vi "error_handler.vi"(7 "calling_vi":refnum<vi>, 8 "error in (no error)":errorcluster, 10 "ni.com link visible (F)":bool, 11 "type of dialog (OK msg:1)":T1=enum."OK message") -> (0 "error out":errorcluster)   [LabVIEW 2015, in "lv-dialog.lvlib"]
doc: "Indicates whether an error occurred. If an error occurred, this VI returns a description of the error and optionally displays a dialog box."
uses:
  lv-dialog.lvlib
  <vilib>/Utility/error.llb/DialogTypeEnum.ctl
  <vilib>/Utility/error.llb/whitespace.ctl
  api/v1/public/_controls/selection.ctl
  api/v1/public/class/v1.lvclass
  api/v1/v1.lvlib
panel:
  # "reinitialize to default to display instructions"
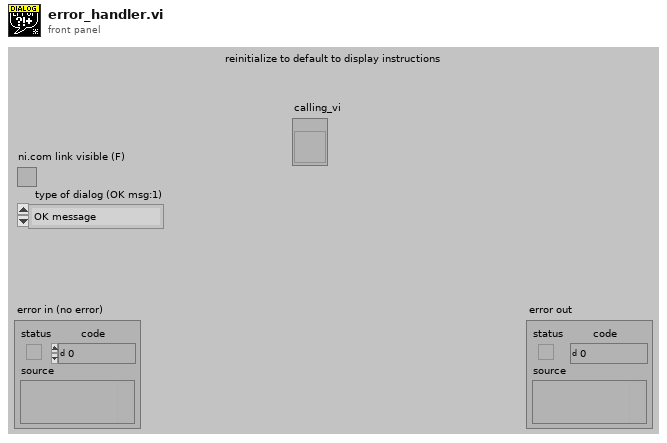
[diagram p1: front panel]
types:
  T1 = typedef "DialogTypeEnum.ctl" = enum16{"no dialog", "OK message", "continue or stop message", "auto error handling dialog", "OK message + warnings", "continue/stop + warnings"}
  T2 = cluster{"Error %d occurred at %s":string, "Warning %d occurred at %s":string, "Possible reasons: %s":string, "Error not listed":string, "GetCommError x%lx":string, "Continue":string, "Stop":string, "an unidentified location":string, "No Error":string, "Help":string}
  T3 = typedef "lv-dialog.lvlib/v1.lvlib/selection.ctl" = enum16{"null", "panel_closed", "button_1", "button_2", "button_3", "cancelled"}
  T4 = typedef "TagReturnType.ctl" = enum16{"No Tag", "<err>", "<append>"}
  T5 = typedef "whitespace.ctl" = u16
  T6 = cluster{"message":string, "Continue":string, "Stop":string}
  T7 = cluster{"ni.com link visible (F)":bool, "code":i32, "Bold Length":i32[], "Bold Start":i32[], "Source Out":string, "Details Out":string, "type of dialog (OK msg:1)":T1, bool, "Continue":string, "Stop":string, "Continue":string, "Tag Found?":T4}
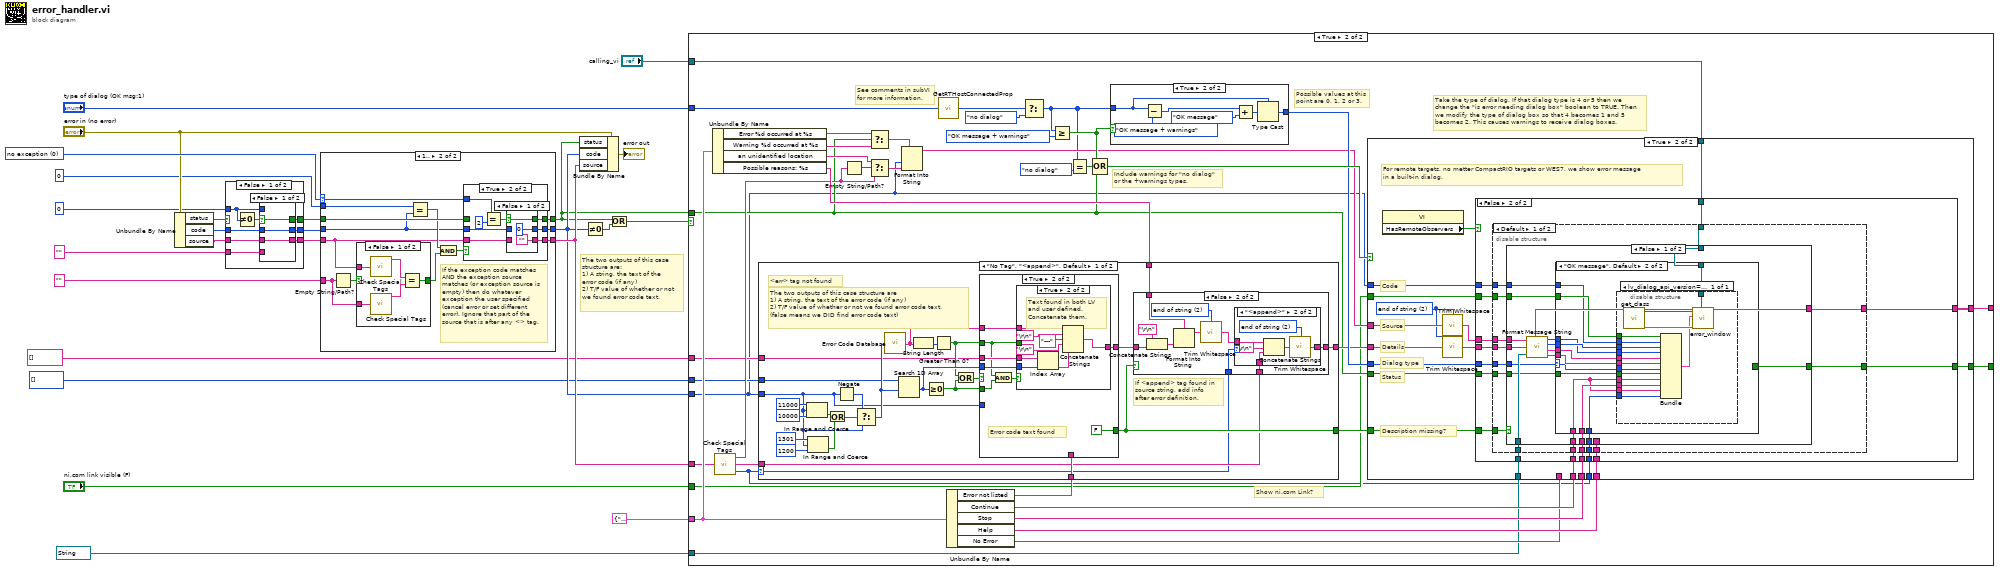
[diagram p0: block diagram]
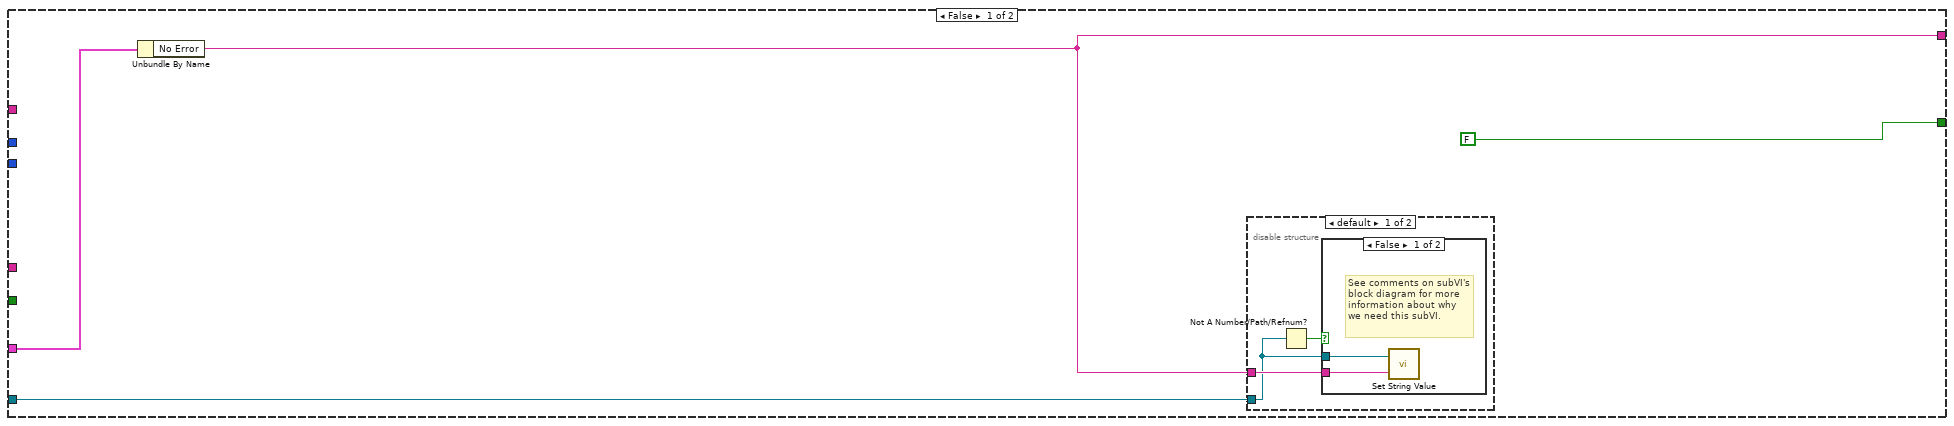
[diagram p8: hidden frame]
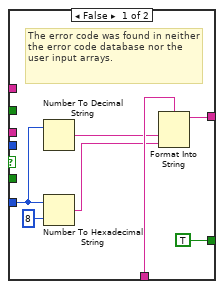
[diagram p14: hidden frame]
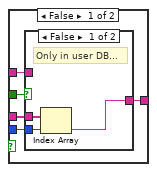
[diagram p15: hidden frame]
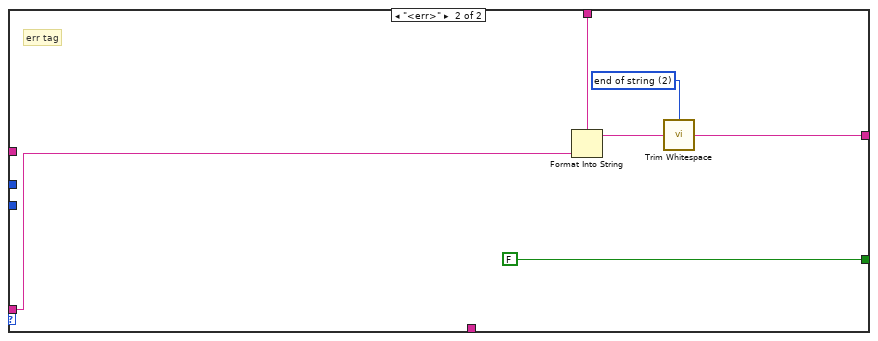
[diagram p17: hidden frame]
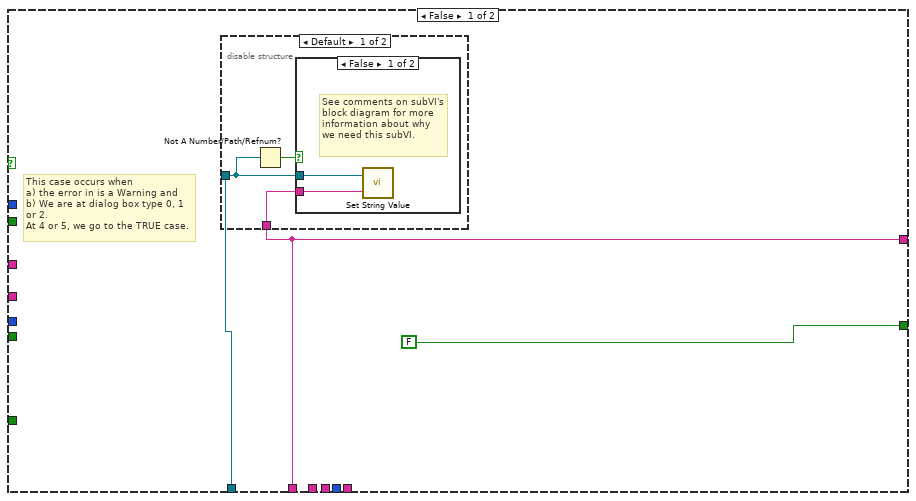
[diagram p18: hidden frame]
diagram:
  w20 = 0 items=["no exception", "cancel error on match", "set error on match"] ("[exception action] (none:0)")
  # "The two outputs of this case structure are:\n1) A string, the text of the error code (if any)\n2) T/F value of whether or not we found error code text."
  n1 = Unbundle By Name("error in (no error)") -> ("status"=w8:bool, "code"=w21:i32, "source"=w25:string)
  n2 = case shown="False" w8 {
    selector: w8 -> [_ w42]
    tunnel: [w31 w41] -> w23
    tunnel: [w32 w42] -> w22
    tunnel: w21 -> [w28 w41]
    tunnel: [w30 w40] -> w24
    tunnel: w25 -> [w29 w40]
    tunnel: 0 ("[error code] (0)") -> [w27 _]
    tunnel: "" ("[error source] (\" \")") -> [w26 _]
    frame False {
      n3 = Not Equal To 0?(x=w27) -> (x != 0?=w33:bool)
      n4 = case shown="False" w33 {
        selector: w33 -> [w36 w39]
        tunnel: [w36 w39] -> w32
        tunnel: w27 -> [_ w38]
        tunnel: [w34 w38] -> w31
        tunnel: w26 -> [_ w37]
        tunnel: [w35 w37] -> w30
        tunnel: w29 -> [w35 _]
        tunnel: w28 -> [w34 _]
        frame False {
        }
        frame True {
        }
      }
    }
    frame True {
    }
  }
  n5 = case shown="1.." w20 {
    selector: w20 -> [_ w50]
    tunnel: [w45 w58] -> w4
    tunnel: w22 -> [w45 w56]
    tunnel: [w44 w57] -> w9
    tunnel: w23 -> [w44 w54]
    tunnel: [w43 w52] -> w18
    tunnel: w24 -> [w43 w48]
    tunnel: 0 ("[exception code]") -> [_ w51]
    tunnel: "" ("[exception source]") -> [_ w47]
    frame ..0 {
    }
    frame 1.. {
      # "If the exception code matches AND the exception source matches (or exception source is empty) then do whatever exception the user specified (cancel error or set different error). Ignore that part of the source that is after any <> tag."
      n6 = Empty String/Path?(string/path=w47) -> (empty?=w49:bool)
      n7 = case shown="False" w49 {
        selector: w49 -> [_ w64]
        tunnel: w48 -> [w63 _]
        tunnel: w47 -> [w62 _]
        tunnel: [w61 w64] -> w46
        frame False {
          n8 = call <vilib>:"Check Special Tags.vi"("source"=w63) -> ("Before Tag (source)"=w60:string)  [unwired: 2 out]
          n9 = call <vilib>:"Check Special Tags.vi"("source"=w62) -> ("Before Tag (source)"=w59:string)  [unwired: 2 out]
          n10 = Equal?(x=w60, y=w59) -> (x = y?=w61:bool)
        }
        frame True {
          # "Empty string always matches."
        }
      }
      n11 = Equal?(x=w51, y=w54) -> (x = y?=w55:bool)
      n12 = And(x=w55, y=w46) -> (x .and. y?=w53:bool)
      n13 = case shown="True" w53 {
        tunnel: [w67 w68] -> w58
        tunnel: [w66 w72] -> w57
        tunnel: w56 -> [w67 _]
        tunnel: w54 -> [w66 w71]
        tunnel: w50 -> [_ w75]
        tunnel: [w65 w70] -> w52
        tunnel: w48 -> [w65 w69]
        frame False {
        }
        frame True {
          n14 = Equal?(x=w75, y=2) -> (x = y?=w73:bool)
          n15 = case shown="False" w73 {
            selector: w73 -> [w78 w81]
            tunnel: [0 w80] -> w72
            tunnel: w71 -> [_ w80]
            tunnel: ["" ("Empty String Constant") w79] -> w70
            tunnel: w69 -> [_ w79]
            tunnel: [w78 w81] -> w68
            frame False {
            }
            frame True {
            }
          }
        }
      }
    }
  }
  n16 = Bundle By Name(cluster="error in (no error)", "status"=w4, "code"=w9, "source"=w18) -> (→"error out":errorcluster)
  n17 = Not Equal To 0?(x=w9) -> (x != 0?=w3:bool)
  n18 = Or(x=w4, y=w3) -> (x .or. y?=w19:bool)
  n19 = case shown="True" w19 {
    tunnel: [w83 w112] -> _
    tunnel: w4 -> [_ w95]
    tunnel: w18 -> [_ w102]
    tunnel: T2 {"Error %d occurred at %s"="Error %d occurred at %s", "Warning %d occurred at %s"="Warning %d occurred at %s", "Possible reasons: %s"="<b>Possible reason(s):</b>\\n%s", "Error not listed"="This error code is undefined. Undefined errors might occur for a number of reasons. For example, no one has provided a description for the code, or you might have wired a number that is not an error code to the error code input. \n\nAdditionally, undefined error codes might occur because the error relates to a third-party object, such as the operating system or ActiveX. For these third-party errors, you might be able to obtain a description of the error by searching the Web for the error code (%s) or for its hexadecimal representation (0x%s).", "GetCommError x%lx"="Windows GetCommError:  The hex value of this code is <B>x%04lx</B>.\n\nInterpret it bit-wise as follows:\n<B>x4000</B>: serial port VI error\n<B>x0001</B>: receiving queue overflowed or character was received after end-of-file character\n<B>x0002</B>: character was lost by overwrite\n<B>x0004</B>: parity error\n<B>x0008</B>: framing error\n<B>x0010</B>: break condition\n<B>x0020</B>: CTS timeout\n<B>x0040</B>: DSR timeout\n<B>x0080</B>: RLSD timeout\n<B>x0100</B>: transmission queue was full when new character arrived\n<B>x0200</B>: parallel device timeout\n<B>x0400</B>: parallel device I/O error\n<B>x0800</B>: parallel device not selected\n<B>x1000</B>: parallel device out of paper\n<B>x8000</B>: requested mode is  not supported or the idComDev parameter is invalid.", "Continue"="Continue", "Stop"="Stop", "an unidentified location"="an unidentified location", "No Error"="No Error", "Help"="Why not found?"} ("prompts") -> [w85 w120]
    tunnel: [FALSE ("Stop 2") w115] -> _
    tunnel: refnum<vi> refnum ("String to Format (not a refnum)") -> [w82 w108]
    tunnel: w9 -> [_ w93]
    tunnel: string[] [] ("[user-defined descriptions]") -> [_ w99]
    tunnel: i32[] [] ("[user-defined codes]") -> [_ w98]
    tunnel: "type of dialog (OK msg:1)" -> [_ w97]
    tunnel: "ni.com link visible (F)" -> [_ w94]
    tunnel: "calling_vi" -> [_ w91]
    frame False {
      n20 = Unbundle By Name(w85) -> ("No Error"=w83:string)
      n21 = disable-structure shown="default" {
        disable-tunnel: w83 -> [w88 _]
        disable-tunnel: w82 -> [w87 _]
        frame condition #0 (active) {
          n22 = Not A Number/Path/Refnum?(number/path/refnum=w87) -> (NaN/Path/Refnum?=w86:bool)
          n23 = case shown="False" w86 {
            tunnel: w88 -> [w90 _]
            tunnel: w87 -> [w89 _]
            frame False {
              # "See comments on subVI's block diagram for more information about why we need this subVI."
              n24 = call <vilib>:"Set String Value.vi"("No Error"=w90, "String to Format (not a refnum)"=w89) -> ()
            }
            frame True {
            }
          }
        }
        frame condition #1 {
          # "Do nothing in RT case."
        }
      }
    }
    frame True {
      # "Show ni.com Link?"
      # "See comments in subVI for more information."
      # "Include warnings for \"no dialog\" or the +warnings types."
      # "Possible values at this point are 0, 1, 2 or 3."
      # "Take the type of dialog. If that dialog type is 4 or 5 then we change the \"is error needing dialog box\" boolean to TRUE. Then we modify the type of dialog box so that 4 becomes 1 and 5 becomes 2. This causes warnings to receive dialog boxes."
      n25 = Unbundle By Name(w120) -> ("Error %d occurred at %s"=w100:string, "Warning %d occurred at %s"=w127:string, "an unidentified location"=w124:string, "Possible reasons: %s"=w114:string)
      n26 = call <vilib>:"Check Special Tags.vi"("source"=w102) -> ("Before Tag (source)"=w101:string, "After Tag (special data)"=w128:string, "Tag Found?"=w92:T4)
      n27 = Empty String/Path?(string/path=w101) -> (empty?=w129:bool)
      n28 = Select(t=w100, s=w95, f=w127) -> (s? t:f=w126:string)
      n29 = Select(t=w124, s=w129, f=w101) -> (s? t:f=w125:string)
      n30 = Format Into String(format string=w126, w93, w125) -> (resulting string=w110:string)  [unwired: 2 in, 1 out]
      n31 = call <vilib>:"GetRTHostConnectedProp.vi"() -> ("App.RTHostConnected"=w96:bool)
      n32 = Unbundle By Name(w120) -> ("Error not listed"=w123:string, "Continue"=w122:string, "Stop"=w121:string, "Help"=w118:string, "No Error"=w109:string)
      n33 = case shown="\"No Tag\", \"<append>\", Default" w92 {
        selector: w92 -> [w137 _]
        tunnel: [w142 w215] -> w111
        tunnel: w93 -> [w138 _]
        tunnel: w128 -> [w143 w214]
        tunnel: w123 -> [w161 _]
        tunnel: [w144 FALSE] -> w119
        tunnel: w114 -> [w146 w213]
        tunnel: w99 -> [w140 _]
        tunnel: w98 -> [w139 _]
        frame "No Tag", "<append>", Default {
          # "If <append> tag found in source string, add info after error definition."
          # "<err> tag not found"
          # "The two outputs of this case structure are\n1) A string, the text of the error code (if any)\n2) T/F value of whether or not we found error code text.\n(false means we DID find error code text)"
          n34 = In Range and Coerce(upper limit=11000, x=w138, lower limit=10000) -> (In Range?=w154:bool)  [unwired: 1 out]
          n35 = In Range and Coerce(upper limit=1301, x=w138, lower limit=1200) -> (In Range?=w155:bool)  [unwired: 1 out]
          n36 = Or(x=w154, y=w155) -> (x .or. y?=w153:bool)
          n37 = Negate(x=w138) -> (-x=w157:i32)
          n38 = Select(t=w157, s=w153, f=w138) -> (s? t:f=w141:i32)
          n39 = call <vilib>:"Error Code Database.vi"("Error Code"=w141) -> ("Error Text"=w147:string)
          n40 = Search 1D Array(1D array=w139, element=w141) -> (index of element=w160:i32)  [unwired: 1 in]
          n41 = String Length(string=w147) -> (length=w151:i32)
          n42 = Greater Or Equal To 0?(x=w160) -> (x >= 0?=w148:bool)
          n43 = Greater Than 0?(x=w151) -> (x > 0?=w149:bool)
          n44 = Or(x=w149, y=w148) -> (x .or. y?=w150:bool)
          n45 = case shown="True" w150 {
            tunnel: w160 -> [_ w190]
            tunnel: [w184 w188] -> w145
            tunnel: w161 -> [w183 _]
            tunnel: [TRUE FALSE] -> w144
            tunnel: w149 -> [_ w187]
            tunnel: w148 -> [_ w192]
            tunnel: w140 -> [_ w191]
            tunnel: w147 -> [_ w189]
            tunnel: w138 -> [w180 _]
            frame False {
              # "The error code was found in neither the error code database nor the user input arrays."
              n46 = Number To Decimal String(number=w180) -> (decimal integer string=w181:string)  [unwired: 1 in]
              n47 = Number To Hexadecimal String(1:i16 8 ("width (-)"), 2:w180) -> (0:w182:string)
              n48 = Format Into String(format string=w183, w181, w182) -> (resulting string=w184:string)  [unwired: 2 in, 1 out]
            }
            frame True {
              # "Error code text found"
              n49 = And(x=w187, y=w192) -> (x .and. y?=w193:bool)
              n50 = case shown="True" w193 {
                tunnel: w191 -> [w196 w211]
                tunnel: w190 -> [w195 w210]
                tunnel: w189 -> [w197 w204]
                tunnel: [w198 w208] -> w188
                tunnel: w187 -> [w199 _]
                frame False {
                  n51 = case shown="False" w199 {
                    tunnel: [w200 w203] -> w198
                    tunnel: w197 -> [_ w203]
                    tunnel: w196 -> [w202 _]
                    tunnel: w195 -> [w201 _]
                    frame False {
                      # "Only in user DB..."
                      n52 = Index Array(array=w202, index=w201) -> (element=w200:string)
                    }
                    frame True {
                      # "Only in LV DB..."
                    }
                  }
                }
                frame True {
                  # "Text found in both LV\nand user defined. \nConcatenate them."
                  n53 = Index Array(array=w211, index=w210) -> (element=w209:string)
                  n54 = Concatenate Strings(w204, "\r\n" ("End of Line Constant"), "---" ("string"), "\r\n" ("End of Line Constant"), w209) -> (w208:string)
                }
              }
            }
          }
          n55 = case shown="False" w144 {
            tunnel: w146 -> [_ w172]
            tunnel: [w162 w164] -> w142
            tunnel: w145 -> [w162 w169]
            tunnel: w137 -> [_ w166]
            tunnel: w143 -> [_ w165]
            frame True {
              # "no explanation given for error."
            }
            frame False {
              w163 = T5 2 items=["both", "start of string", "end of string"] ("location (both)")
              n56 = Concatenate Strings("\r\n" ("End of Line Constant"), w169) -> (w170:string)
              n57 = Format Into String(format string=w172, w170) -> (resulting string=w171:string)  [unwired: 2 in, 1 out]
              n58 = call <vilib>:"Trim Whitespace.vi"("string"=w171, "location (both)"=w163) -> ("trimmed string"=w167:string)
              n59 = case shown="\"<append>\"" w166 {
                tunnel: w167 -> [w173 w178]
                tunnel: [w173 w175] -> w164
                tunnel: w165 -> [_ w177]
                frame "No Tag", Default {
                }
                frame "<append>" {
                  w174 = T5 2 items=["both", "start of string", "end of string"] ("location (both)")
                  n60 = Concatenate Strings(w178, "\r\n" ("End of Line Constant"), w177) -> (w176:string)
                  n61 = call <vilib>:"Trim Whitespace.vi"("string"=w176, "location (both)"=w174) -> ("trimmed string"=w175:string)
                }
              }
            }
          }
        }
        frame "<err>" {
          w212 = T5 2 items=["both", "start of string", "end of string"] ("location (both)")
          # "err tag"
          n62 = Format Into String(format string=w213, w214) -> (resulting string=w216:string)  [unwired: 2 in, 1 out]
          n63 = call <vilib>:"Trim Whitespace.vi"("string"=w216, "location (both)"=w212) -> ("trimmed string"=w215:string)
        }
      }
      n64 = Select(t=w97, s=w96, f=DialogTypeEnum."no dialog" ("type of dialog (OK msg:1)")) -> (s? t:f=w103:T1)
      n65 = Greater Or Equal?(x=w103, y=DialogTypeEnum."OK message + warnings" ("type of dialog (OK msg:1)")) -> (x >= y?=w116:bool)
      n66 = Equal?(x=w103, y=DialogTypeEnum."no dialog" ("type of dialog (OK msg:1)")) -> (x = y?=w107:bool)
      n67 = Compound Arithmetic op=OR(w116, w107, w95) -> (w117:bool)
      n68 = case shown="True" w116 {
        tunnel: w103 -> [w130 w131]
        tunnel: [w130 w133] -> w113
        frame False {
        }
        frame True {
          n69 = Subtract(x=w131, y=DialogTypeEnum."OK message + warnings" ("type of dialog (OK msg:1)")) -> (x-y=w136:u16)
          n70 = Add(x=w136, y=DialogTypeEnum."OK message" ("type of dialog (OK msg:1)")) -> (x+y=w132:u16)
          n71 = Type Cast(type=w131, x=w132) -> (*(type *) &x=w133:T1)
        }
      }
      n72 = case shown="True" w117 {
        tunnel: w113 -> [_ w244]
        tunnel: w122 -> [_ w243]
        tunnel: w121 -> [_ w242]
        tunnel: w119 -> [_ w231]
        tunnel: w118 -> [_ w241]
        tunnel: w110 -> [_ w234]
        tunnel: w111 -> [_ w235]
        tunnel: w95 -> [_ w240]
        tunnel: [FALSE ("Stop 2") w239] -> w115
        tunnel: [w218 w238] -> w112
        tunnel: w109 -> [w218 _]
        tunnel: w108 -> [w219 w237]
        tunnel: w94 -> [_ w229]
        tunnel: w93 -> [_ w230]
        tunnel: w92 -> [_ w228]
        tunnel: w91 -> [_ w226]
        frame False {
          # "This case occurs when\na) the error in is a Warning and\nb) We are at dialog box type 0, 1 or 2.\nAt 4 or 5, we go to the TRUE case."
          n73 = disable-structure shown="Default" {
            disable-tunnel: w219 -> [w223 _]
            disable-tunnel: w218 -> [w221 _]
            frame condition #0 (active) {
              n74 = Not A Number/Path/Refnum?(number/path/refnum=w223) -> (NaN/Path/Refnum?=w222:bool)
              n75 = case shown="False" w222 {
                tunnel: w221 -> [w225 _]
                tunnel: w223 -> [w224 _]
                frame False {
                  # "See comments on subVI's block diagram for more information about why we need this subVI."
                  n76 = call <vilib>:"Set String Value.vi"("No Error"=w225, "String to Format (not a refnum)"=w224) -> ()
                }
                frame True {
                }
              }
            }
            frame condition #1 {
              # "Do nothing in RT case."
            }
          }
        }
        frame True {
          w232 = T5 2 items=["both", "start of string", "end of string"] ("location (both)")
          # "For remote targets, no metter CompactRIO targets or WES7, we show error message \nin a built-in dialog."
          # "Code"
          # "Description missing?"
          # "Dialog type"
          # "Status"
          # "Details"
          # "Source"
          n77 = property class="VI"() -> ("HasRemoteObservers"=w227:bool)  [unwired: 2 in, 2 out]
          n78 = call <vilib>:"Trim Whitespace.vi"("string"=w234, "location (both)"=w232) -> ("trimmed string"=w233:string)
          n79 = call <vilib>:"Trim Whitespace.vi"("string"=w235, "location (both)"=w232) -> ("trimmed string"=w236:string)
          n80 = case shown="False" w227 {
            tunnel: w244 -> [w246 w305]
            tunnel: w243 -> [w250 w304]
            tunnel: w242 -> [w249 w303]
            tunnel: w241 -> [_ w302]
            tunnel: w240 -> [_ w301]
            tunnel: [w248 w300] -> w239
            tunnel: [w247 w299] -> w238
            tunnel: w237 -> [w251 w298]
            tunnel: w236 -> [w252 w297]
            tunnel: w233 -> [w253 w296]
            tunnel: w231 -> [_ w295]
            tunnel: w230 -> [_ w294]
            tunnel: w229 -> [_ w293]
            tunnel: w228 -> [_ w292]
            tunnel: w226 -> [w245 w291]
            frame True {
              n81 = call <vilib>:"Format Message String.vi"("Source"=w253, "Details"=w252, "String to Format (not a refnum)"=w251) -> ("message"=w247:string)  [unwired: 1 in, 4 out]
              n82 = disable-structure shown="lv_dialog_api_version==1, Default" {
                disable-tunnel: w250 -> [w261]
                disable-tunnel: w249 -> [w260]
                disable-tunnel: [w259] -> w248
                disable-tunnel: w247 -> [w258]
                disable-tunnel: w246 -> [w257]
                disable-tunnel: w245 -> [w256]
                frame condition #0 (active) {
                  n83 = call "get_class.vi"() -> ("error out"=w254:errorcluster, "class"=w255:refnum<class "v1.lvclass">)  [unwired: 10 in]
                  n84 = case shown="\"OK message\", \"OK message + warnings\", Default" w257 {
                    tunnel: [FALSE ("stop event propagated") FALSE ("stop event propagated") FALSE w287] -> w259
                    tunnel: w258 -> [_ w267 w278 w286]
                    tunnel: w261 -> [_ w266 w277 w285]
                    tunnel: w260 -> [_ _ w273 w284]
                    tunnel: w256 -> [_ w268 w272 w283]
                    tunnel: w255 -> [_ w263 w271 w282]
                    tunnel: w254 -> [_ w264 w270 w281]
                    frame "no dialog" {
                    }
                    frame "OK message", "OK message + warnings", Default {
                      n85 = Bundle("message"=w267, "Continue"=w266) -> (w265:cluster{"message":string, "Continue":string})  [unwired: 1 in]
                      n86 = call-dynamic "one_button.vi"("callee"=w268, "error in (no error)"=w264, "configuration"=w265, "v1 in"=w263) -> ()  [unwired: 5 in, 3 out]
                    }
                    frame "continue or stop message", "continue/stop + warnings" {
                      n87 = Bundle("message"=w278, "Continue"=w277, "Stop"=w273) -> (w274:T6)  [unwired: 1 in]
                      n88 = call-dynamic "two_button.vi"("callee"=w272, "error in (no error)"=w270, "configuration"=w274, "v1 in"=w271) -> ("dialog_selection"=w280:T3)  [unwired: 5 in, 2 out]
                      n89 = Equal?(x=w280, y=selection."button_2") -> (x = y?=w276:bool)
                      n90 = Stop(stop? (T)=w276) -> ()
                    }
                    frame "auto error handling dialog" {
                      n91 = Bundle("message"=w286, "Continue"=w285, "Stop"=w284) -> (w288:T6)  [unwired: 1 in]
                      n92 = call-dynamic "two_button.vi"("callee"=w283, "error in (no error)"=w281, "configuration"=w288, "v1 in"=w282) -> ("dialog_selection"=w290:T3)  [unwired: 5 in, 2 out]
                      n93 = Equal?(x=w290, y=selection."button_2") -> (x = y?=w287:bool)
                    }
                  }
                }
              }
            }
            frame False {
              n94 = disable-structure "Conditional Disable Structure" shown="Default" {
                disable-tunnel: w305 -> [w320 _]
                disable-tunnel: w304 -> [w319 _]
                disable-tunnel: w303 -> [w318 _]
                disable-tunnel: w302 -> [w317 _]
                disable-tunnel: w301 -> [w316 _]
                disable-tunnel: [w315 FALSE ("stop event propagated")] -> w300
                disable-tunnel: [w314 w380] -> w299
                disable-tunnel: w298 -> [w313 w381]
                disable-tunnel: w297 -> [w312 w382]
                disable-tunnel: w296 -> [w311 w383]
                disable-tunnel: w295 -> [w310 _]
                disable-tunnel: w293 -> [w308 _]
                disable-tunnel: w294 -> [w309 _]
                disable-tunnel: w292 -> [w307 _]
                disable-tunnel: w291 -> [w306 _]
                frame condition #0 (active) {
                  n95 = case shown="False" w310 {
                    tunnel: w312 -> [w336 w371]
                    tunnel: w317 -> [_ w377]
                    tunnel: w319 -> [w332 w375]
                    tunnel: w318 -> [w331 w374]
                    tunnel: w320 -> [w334 w376]
                    tunnel: [w333 w373] -> w315
                    tunnel: w311 -> [w337 w372]
                    tunnel: w316 -> [w330 _]
                    tunnel: [w325 w369] -> w314
                    tunnel: w313 -> [w335 w367]
                    tunnel: w308 -> [w323 _]
                    tunnel: w309 -> [w324 _]
                    tunnel: w307 -> [w322 _]
                    tunnel: w306 -> [w321 _]
                    frame False {
                      n96 = call <vilib>:"Format Message String.vi"("Source"=w337, "Details"=w336, "String to Format (not a refnum)"=w335) -> ("message"=w325:string, "Bold Start"=w329:i32[], "Bold Length"=w328:i32[], "Source Out"=w327:string, "Details Out"=w326:string)  [unwired: 1 in]
                      n97 = case shown="\"OK message\", Default" w334 {
                        selector: w334 -> [_ w343]
                        tunnel: [FALSE ("stop event propagated") _] -> w333
                        tunnel: w332 -> [_ w340]
                        tunnel: w331 -> [_ w341]
                        tunnel: w330 -> [_ w342]
                        tunnel: w329 -> [_ w346]
                        tunnel: w328 -> [_ w347]
                        tunnel: w327 -> [_ w345]
                        tunnel: w326 -> [_ w344]
                        tunnel: w323 -> [_ w349]
                        tunnel: w324 -> [_ w348]
                        tunnel: w322 -> [_ w339]
                        tunnel: w321 -> [_ w350]
                        frame "no dialog" {
                        }
                        frame "OK message", Default {
                          n98 = disable-structure shown="lv_dialog_api_version==1, Default" {
                            disable-tunnel: w350 -> [w366]
                            disable-tunnel: w349 -> [w362]
                            disable-tunnel: w348 -> [w361]
                            disable-tunnel: w347 -> [w360]
                            disable-tunnel: w346 -> [w359]
                            disable-tunnel: w345 -> [w358]
                            disable-tunnel: w344 -> [w357]
                            disable-tunnel: w343 -> [w356]
                            disable-tunnel: w342 -> [w355]
                            disable-tunnel: w340 -> [w354]
                            disable-tunnel: w341 -> [w353]
                            disable-tunnel: w340 -> [w352]
                            disable-tunnel: w339 -> [w351]
                            frame condition #0 (active) {
                              n99 = call "get_class.vi"() -> ("error out"=w364:errorcluster, "class"=w365:refnum<class "v1.lvclass">)  [unwired: 10 in]
                              n100 = Bundle("ni.com link visible (F)"=w362, "code"=w361, "Bold Length"=w360, "Bold Start"=w359, "Source Out"=w358, "Details Out"=w357, "type of dialog (OK msg:1)"=w356, w355, "Continue"=w354, "Stop"=w353, "Continue"=w352, "Tag Found?"=w351) -> (w363:T7)  [unwired: 1 in]
                              n101 = call-dynamic "error_window.vi"("callee"=w366, "error in (no error)"=w364, "configuration"=w363, "v1 in"=w365) -> ()  [unwired: 5 in, 3 out]
                            }
                          }
                        }
                      }
                    }
                    frame True {
                      w370 = "\r\n" ("End of Line Constant")
                      n102 = Concatenate Strings(w372, w370, w370, w371) -> (w369:string)
                      n103 = Not A Number/Path/Refnum?(number/path/refnum=w367) -> (NaN/Path/Refnum?=w368:bool)
                      n104 = call <vilib>:"Not Found Dialog.vi"("Help"=w377, "Message"=w369, "Stop"=w374, "Continue"=w375, "type of dialog (OK msg:1)"=w376) -> ("stop event propagated"=w373:bool)  [unwired: 1 in]
                      n105 = case shown="True" w368 {
                        tunnel: w367 -> [w379 _]
                        tunnel: w369 -> [w378 _]
                        frame False {
                          n106 = call <vilib>:"Set String Value.vi"("No Error"=w378, "String to Format (not a refnum)"=w379) -> ()
                        }
                        frame True {
                        }
                      }
                    }
                  }
                }
                frame condition #1 {
                  n107 = call <vilib>:"Format Message String.vi"("Source"=w383, "Details"=w382, "String to Format (not a refnum)"=w381) -> ("message"=w380:string)  [unwired: 1 in, 4 out]
                }
              }
            }
          }
        }
      }
    }
  }
